vi "Poly2Bounds.vi"(10 "Border":dbl, 11 "Polys":T2[](array[typedef])) -> (3 "Bounds":T1)   [LabVIEW 2014]
uses:
  TypeDefs/Poly2DwSlope.ctl
  TypeDefs/Point2DwSlope.ctl
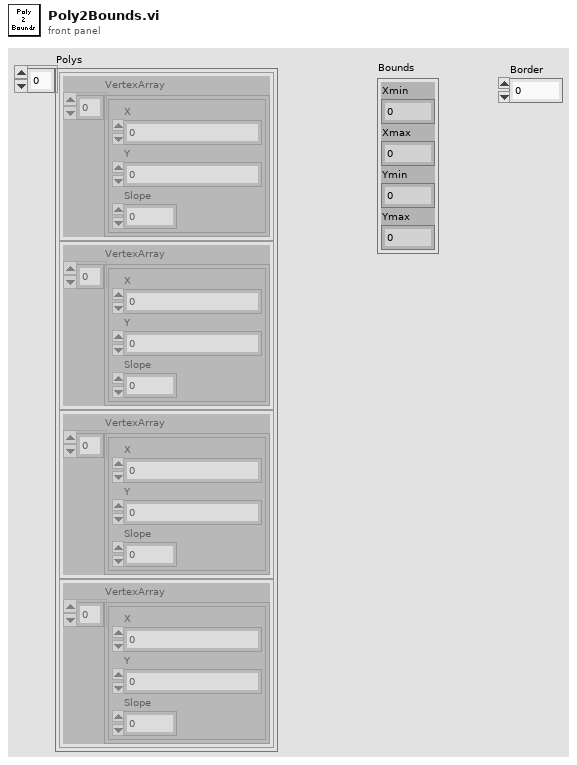
[diagram p1: front panel]
types:
  T1 = cluster{"Xmin":dbl, "Xmax":dbl, "Ymin":dbl, "Ymax":dbl}
  T2 = typedef "Poly2DwSlope.ctl" = cluster{"VertexArray":T3[]}
  T3 = typedef "Point2DwSlope.ctl" = cluster{"X":sgl, "Y":sgl, "Slope":dbl}
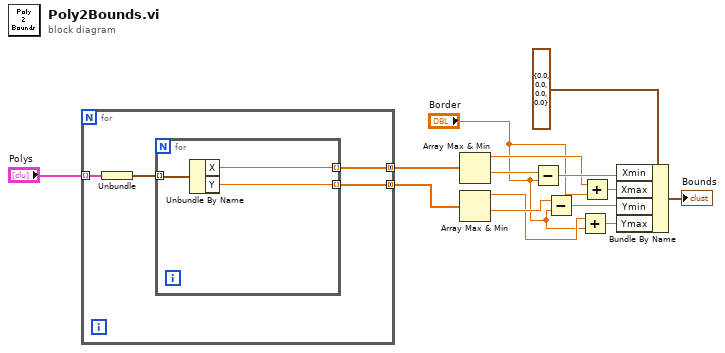
[diagram p0: block diagram]
diagram:
  n1 = for {
    tunnel: "Polys" -> [w18] mode=indexing
    tunnel: [w16] -> w13 mode=concatenating
    tunnel: [w15] -> w12 mode=concatenating
    n2 = Unbundle(w18) -> ("VertexArray"=w17:T3[])
    n3 = for {
      tunnel: w17 -> [w21] mode=indexing
      tunnel: [w20] -> w16 mode=indexing
      tunnel: [w19] -> w15 mode=indexing
      n4 = Unbundle By Name(w21) -> ("X"=w20:sgl, "Y"=w19:sgl)
    }
  }
  n5 = Array Max & Min(array=w13) -> (max value=w7:sgl, min value=w9:sgl)  [unwired: 2 out]
  n6 = Array Max & Min(array=w12) -> (max value=w2:sgl, min value=w4:sgl)  [unwired: 2 out]
  n7 = Subtract(x=w9, y="Border") -> (x-y=w8:dbl)
  n8 = Subtract(x=w4, y="Border") -> (x-y=w5:dbl)
  n9 = Add(x=w2, y="Border") -> (x+y=w3:dbl)
  n10 = Add(x=w7, y="Border") -> (x+y=w6:dbl)
  n11 = Bundle By Name(cluster=T1 {"Xmin"=0.0, "Xmax"=0.0, "Ymin"=0.0, "Ymax"=0.0} ("Bounds"), "Xmin"=w8, "Xmax"=w6, "Ymin"=w5, "Ymax"=w3) -> (→"Bounds":T1)
